vi "Serialize.vi"(8 "error in":errorcluster, 9 "OwningElement in":refnum<k20>, 10 "Document in":refnum<k20>, 11 "Defect in":refnum<class "Defect.lvclass">) -> (0 "error out":errorcluster, 1 "OwningElement out":refnum<k20>, 2 "Document out":refnum<k20>, 3 "Defect out":refnum<class "Defect.lvclass">)   [LabVIEW 2021, in "ProligentXMLGenerator.lvlib" / "Defect.lvclass"]
uses:
  Defect.lvclass
  Defect.lvclass/Defect.ctl
  <vilib>/xml/NI_XML.lvlib
  Model/UserComment/UserComment.lvclass
  Base/DOMSupport/DOMSupport.lvlib
  Model/CustomData/CustomData.lvclass
  <vilib>/xml/Close Reference(Node).vi
  Base/DateTime/DateTime.lvclass
  C:/Projects/proligent-xml-generator-labview/src/ProligentXMLGenerator/Base/Attribute/Attribute.lvclass
  C:/Projects/proligent-xml-generator-labview/src/ProligentXMLGenerator/Base/DateTime/DateTime.lvclass
  Base/Guid/Guid.lvclass
  C:/Projects/proligent-xml-generator-labview/src/ProligentXMLGenerator/Base/NonEmptyString/NonEmptyString.lvclass
  C:/Projects/proligent-xml-generator-labview/src/ProligentXMLGenerator/Base/String/String.lvclass
  C:/Projects/proligent-xml-generator-labview/src/ProligentXMLGenerator/Base/Guid/Guid.lvclass
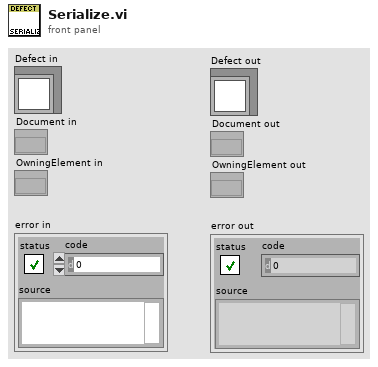
[diagram p1: front panel]
types:
  T1 = typedef "ProligentXMLGenerator.lvlib/Defect.lvclass/Data.ctl" = cluster{"Name":string, "Comments":refnum<class "UserComment.lvclass">[], "CustomData":refnum<class "CustomData.lvclass">, "DefectId":refnum<class "Guid.lvclass">, "OpenTime":refnum<class "DateTime.lvclass">, "TimeZoneInfoId":string}
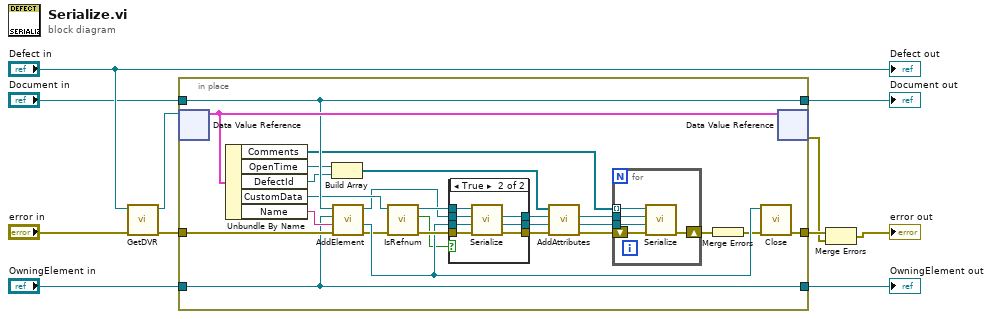
[diagram p0: block diagram]
diagram:
  n1 = call "GetDVR.vi"("error in"="error in", "Defect"="Defect in") -> ("error out"=w3:errorcluster, "DVRReference"=w2:refnum<data-value>)  [unwired: 8 in]
  n2 = in-place "In Place Element Structure" {
    in-place-border: [w36] -> w4
    in-place-border: "Document in" -> [w30]
    in-place-border: w3 -> [w35]
    in-place-border: "OwningElement in" -> [w33]
    in-place-border: [w33] -> w6
    in-place-border: [w30] -> w5
    n3 = in-place-dvr #1(w2) -> (w32:T1)  [unwired: 1 out]
    n4 = Unbundle By Name(w32) -> ("Comments"=w14:refnum<class "UserComment.lvclass">[], "OpenTime"=w24:refnum<class "DateTime.lvclass">, "DefectId"=w23:refnum<class "Guid.lvclass">, "CustomData"=w26:refnum<class "CustomData.lvclass">, "Name"=w34:string)
    n5 = Build Array(w24, w23) -> (w22:refnum<class "Attribute.lvclass">[])
    n6 = call "AddElement.vi"("error in"=w35, "Name"=w34, "OwningElement in"=w33, "Document in"=w30) -> ("error out"=w13:errorcluster, "NewElement"=w28:refnum<k20>, "Document out"=w21:refnum<k20>)  [unwired: 4 in, 1 out]
    n7 = call "IsRefnum.vi"("error in"=w13, "CustomDataType in"=w26) -> ("error out"=w29:errorcluster, "IsRefnum"=w25:bool, "CustomDataType out"=w27:refnum<class "CustomData.lvclass">)  [unwired: 7 in]
    n8 = case shown="True" w25 {
      tunnel: w21 -> [w38 w46]
      tunnel: w29 -> [w39 w45]
      tunnel: w28 -> [w37 w44]
      tunnel: [w39 w43] -> w16
      tunnel: w27 -> [_ w42]
      tunnel: [w38 w41] -> w17
      tunnel: [w37 w40] -> w18
      frame False {
      }
      frame True {
        n9 = call "Serialize.vi"("error in"=w45, "OwningElement in"=w44, "Document in"=w46, "CustomDataType in"=w42) -> ("error out"=w43:errorcluster, "OwningElement out"=w40:refnum<k20>, "Document out"=w41:refnum<k20>)  [unwired: 4 in, 1 out]
      }
    }
    n10 = call "AddAttributes.vi"("error in"=w16, "OwningElement in"=w18, "Document in"=w17, "Attributes"=w22) -> ("error out"=w15:errorcluster, "OwningElement out"=w19:refnum<k20>, "Document out"=w20:refnum<k20>)  [unwired: 5 in]
    n11 = for {
      tunnel: w14 -> [w51] mode=indexing
      tunnel: w19 -> [w49]
      tunnel: w20 -> [w50]
      shift-right: [w47] -> w31
      shift-left: w15 -> [w48]
      n12 = call "Serialize.vi"("error in"=w48, "OwningElement in"=w49, "Document in"=w50, "UserComment in"=w51) -> ("error out"=w47:errorcluster)  [unwired: 4 in, 3 out]
    }
    n13 = Merge Errors(w31) -> (w12:errorcluster)
    n14 = call-poly <vilib>:"Close.vi"("error in (no error)"=w12, "node"=w28) -> ("error out"=w36:errorcluster)  [unwired: 7 in]
    n15 = in-place-dvr #1(w32) -> (w1:errorcluster)  [unwired: 1 out]
  }
  "Document out" <- w5
  "OwningElement out" <- w6
  n16 = Merge Errors(w4, w1) -> (→"error out":errorcluster)
  "Defect out" <- "Defect in"
